vi "project_synthwaveUI.vi"() -> ()   [LabVIEW 2018]
uses:
  <vilib>/sound2/lvsound2.llb/Sampling Mode.ctl
  <vilib>/sound2/lvsound2.llb/Sound Data Format.ctl
  <vilib>/event_ctls.llb/eventvkey.ctl
  <vilib>/sound2/lvsound2.llb/Sound Output Set Volume (Single).vi
  <vilib>/sound2/lvsound2.llb/Sound Output Write (DBL Single).vi
  <vilib>/measure/NI_MABase.lvlib
panel:
  in  "Volume":dbl(knob)=70.40816326530613 scale=0.0..100.0
  in  "Waveform":enum16{"Sine", "Square", "Sawtooth", "Triangle"}(ring)
  out "Generated Sound":waveform(dbl)(graph)
  in  "Keys":T1(radio)=enum."Boolean 1"
  out "Indice":u32
  out "Note Actual":dbl
  in  "?":bool
  in  "Hold Key":bool
  in  "Octave":dbl min=-3.0 max=4.0 step=1.0
  in  "Note Base":dbl=261.626 format="%.2g"
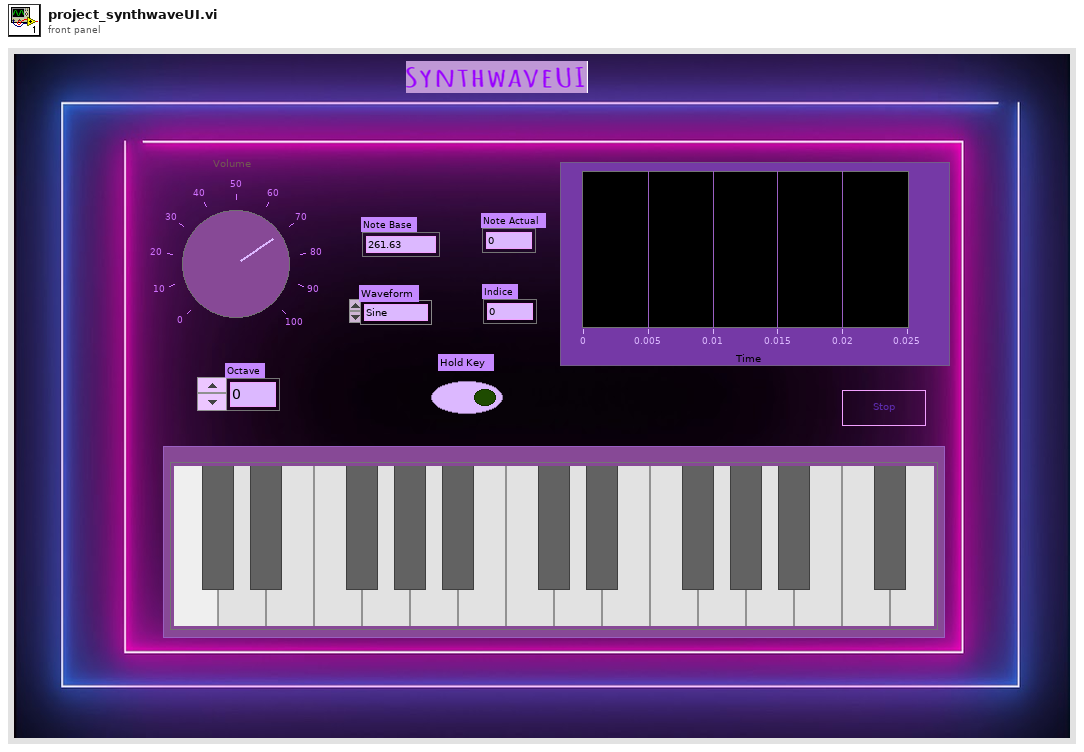
[diagram p1: front panel]
types:
  T1 = enum32{"No Selection", "Boolean 1", "Boolean 2", "Boolean 3", "Boolean 4", "Boolean 5", "Boolean 6", "Boolean 7", "Boolean 8", "Boolean 9", "Boolean 10", "Boolean 11", "Boolean 12", "Boolean 13", "Boolean 14", "Boolean 15", "Boolean 16", "Boolean 17", "Boolean 18", "Boolean 19", "Boolean 20", "Boolean 21", "Boolean 22", "Boolean 23", "Boolean 24", "Boolean 25", "Boolean 26", "Boolean 27"}
  T2 = typedef "eventvkey.ctl" = enum16{"ASCII", "Enter", "Return", "Shift", "Ctrl", "Alt", "Cmd", "Opt", "Caps", "NumLock", "Clear", "Break", "Up", "Down", "Left", "Right", "Insert", "Delete", "Home", "End", "PageUp", "PageDown", "Escape", "Help", "Pause", "ScrollLock", "F1", "F2", "F3", "F4", "F5", "F6", "F7", "F8", "F9", "F10", "F11", "F12", "F13", "F14", "F15", "F16", "F17", "F18", "F19", "F20", "F21", "F22", "F23", "F24", "Play", "VolumeUp", "VolumeDown", "Mute", "Two Byte Char"}
  T3 = typedef "Sound Data Format.ctl" = cluster{"sample rate (S/s)":dbl, "number of channels":i32, "bits per sample":i32}
  T4 = typedef "Sampling Mode.ctl" = i32
  T5 = typedef "Sound Output Task ID.ctl" = u32
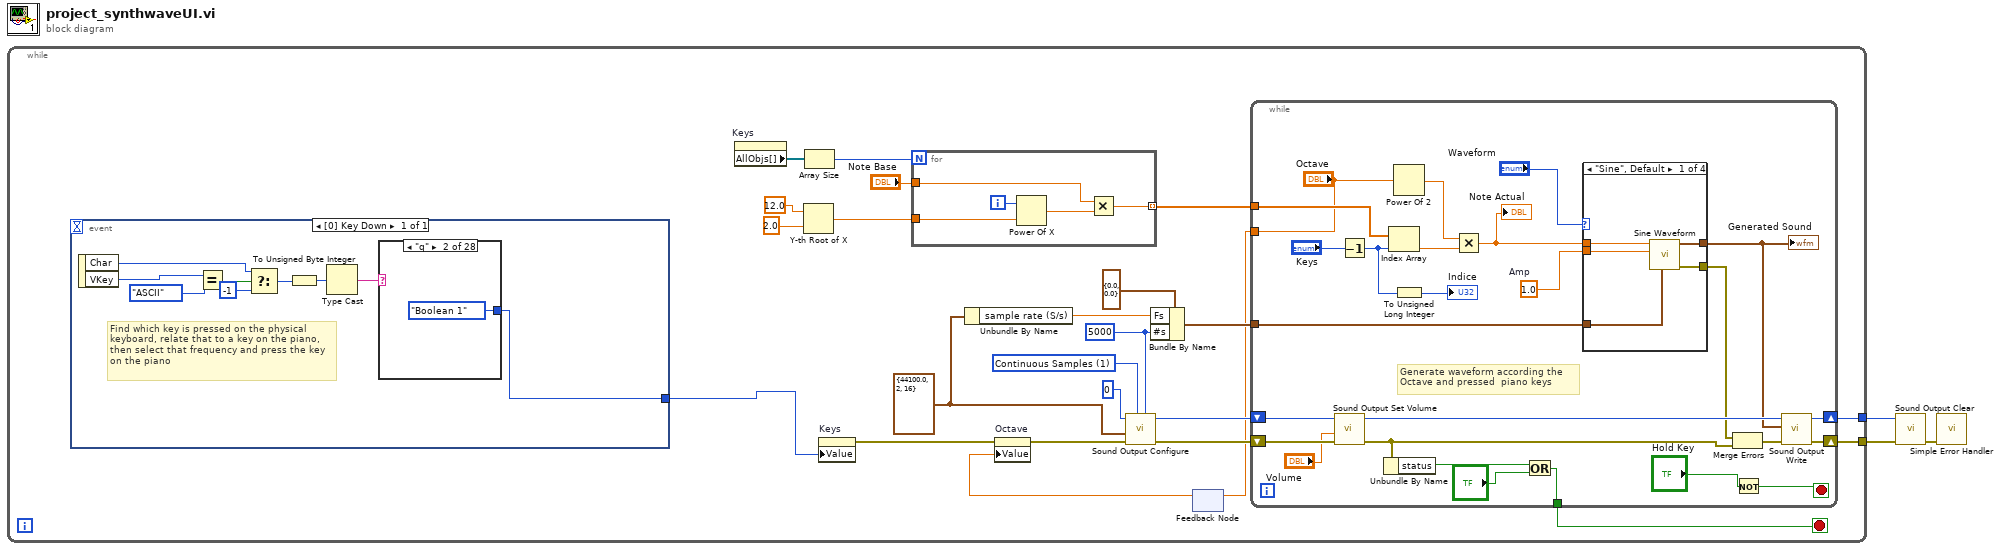
[diagram p0: block diagram]
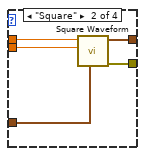
[diagram p2: hidden frame]
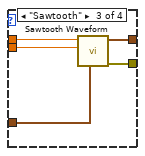
[diagram p3: hidden frame]
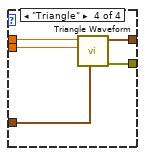
[diagram p4: hidden frame]
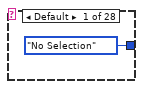
[diagram p5: hidden frame]
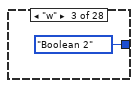
[diagram p6: hidden frame]
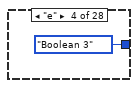
[diagram p7: hidden frame]
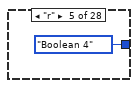
[diagram p8: hidden frame]
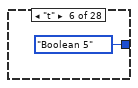
[diagram p9: hidden frame]
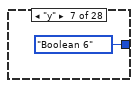
[diagram p10: hidden frame]
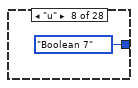
[diagram p11: hidden frame]
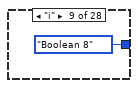
[diagram p12: hidden frame]
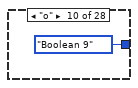
[diagram p13: hidden frame]
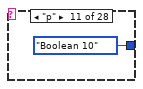
[diagram p14: hidden frame]
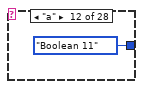
[diagram p15: hidden frame]
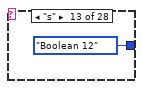
[diagram p16: hidden frame]
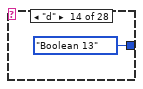
[diagram p17: hidden frame]
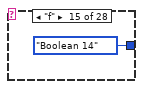
[diagram p18: hidden frame]
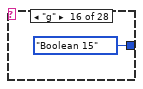
[diagram p19: hidden frame]
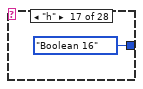
[diagram p20: hidden frame]
diagram:
  n1 = while {
    tunnel: [w27] -> w3
    tunnel: [w26] -> w2
    stop <- w24 stop-if-true
    w12 = 5000 ("Samples/ch")
    w13 = T3 {"sample rate (S/s)"=44100.0, "number of channels"=2, "bits per sample"=16} ("Sound Format")
    w19 = T4 1 items=["Finite Samples", "Continuous Samples"] ("sample mode")
    n2 = event shown="[0] Key Down" {
      selector: _ -> [_]
      dyn-events: _ -> [_]
      timeout: _ -> [_]
      tunnel: [w79] -> w25
      event Key Down {
        # "Find which key is pressed on the physical\nkeyboard, relate that to a key on the piano,\nthen select that frequency and press the key\non the piano"
        n3 = event-data() -> ("Char"=w84:i16, "VKey"=w87:T2)  [unwired: 1 in]
        n4 = Equal?(x=w87, y=eventvkey."ASCII" ("VKey")) -> (x = y?=w85:bool)
        n5 = Select(t=w84, s=w85, f=i16 -1) -> (s? t:f=w81:i16)
        n6 = To Unsigned Byte Integer(number=w81) -> (unsigned 8bit integer=w82:u8)
        n7 = Type Cast(x=w82) -> (*(type *) &x=w80:string)  [unwired: 1 in]
        n8 = case shown="\"q\"" w80 {
          tunnel: [T1."No Selection" ("Keys") T1."Boolean 1" ("Keys") T1."Boolean 2" ("Keys") T1."Boolean 3" ("Keys") T1."Boolean 4" ("Keys") T1."Boolean 5" ("Keys") T1."Boolean 6" ("Keys") T1."Boolean 7" ("Keys") T1."Boolean 8" ("Keys") T1."Boolean 9" ("Keys") T1."Boolean 10" ("Keys") T1."Boolean 11" ("Keys") T1."Boolean 12" ("Keys") T1."Boolean 13" ("Keys") T1."Boolean 14" ("Keys") T1."Boolean 15" ("Keys") T1."Boolean 16" ("Keys") T1."Boolean 17" ("Keys") T1."Boolean 18" ("Keys") T1."Boolean 19" ("Keys") T1."Boolean 20" ("Keys") T1."Boolean 21" ("Keys") T1."Boolean 22" ("Keys") T1."Boolean 23" ("Keys") T1."Boolean 24" ("Keys") T1."Boolean 25" ("Keys") T1."Boolean 26" ("Keys") T1."Boolean 27" ("Keys")] -> w79
          frame Default {
          }
          frame "q" {
          }
          frame "w" {
          }
          frame "e" {
          }
          frame "r" {
          }
          frame "t" {
          }
          frame "y" {
          }
          frame "u" {
          }
          frame "i" {
          }
          frame "o" {
          }
          frame "p" {
          }
          frame "a" {
          }
          frame "s" {
          }
          frame "d" {
          }
          frame "f" {
          }
          frame "g" {
          }
          frame "h" {
          }
          frame "j" {
          }
          frame "k" {
          }
          frame "l" {
          }
          frame ";" {
          }
          frame "z" {
          }
          frame "x" {
          }
          frame "c" {
          }
          frame "v" {
          }
          frame "b" {
          }
          frame "n" {
          }
          frame "m" {
          }
        }
      }
    }
    n9 = property on="Keys" class="RadioBtnsControl (strict)"() -> ("AllObjs[]"=w15:refnum<vi>[])  [unwired: 2 in, 2 out]
    n10 = Y-th Root of X(1:2.0 ("x"), 2:12.0 ("y")) -> (0:w8:dbl)
    n11 = Array Size(array=w15) -> (size(s)=w14:i32)
    n12 = property on="Keys" class="RadioBtnsControl (strict)"("Value"=w25) -> (error out=w7:errorcluster)  [unwired: 2 in, 1 out]
    n13 = for {
      N: w14 -> [_]
      tunnel: [w32] -> w20 mode=indexing
      tunnel: "Note Base" -> [w31]
      tunnel: w8 -> [w28]
      i -> [w30]
      n14 = Power Of X(1:w28, 2:w30) -> (0:w29:dbl)
      n15 = Multiply(x=w31, y=w29) -> (x*y=w32:dbl)
    }
    n16 = Unbundle By Name(w13) -> ("sample rate (S/s)"=w17:dbl)
    n17 = Bundle By Name(cluster=cluster{"Fs":dbl, "#s":dbl} {"Fs"=0.0, "#s"=0.0} ("sampling info"), "Fs"=w17, "#s"=w12) -> (w21:cluster{"Fs":dbl, "#s":dbl})
    n18 = feedback #1() -> (w4:dbl)  [unwired: 1 in]
    n19 = property on="Octave" class="DigNum (strict)"(error in=w7, "Value"=w4) -> (error out=w6:errorcluster)  [unwired: 1 in, 1 out]
    n20 = call <vilib>:"Sound Output Configure.vi"("number of samples/ch"=w12, "sample mode"=w19, "error in (no error)"=w6, "sound format"=w13, "device ID"=u32 0 ("Device ID")) -> ("error out"=w23:errorcluster, "task ID"=w22:T5)  [unwired: 5 in]
    n21 = while {
      tunnel: [w56] -> w24
      tunnel: w21 -> [w53]
      tunnel: w20 -> [w52]
      shift-right: [w58] -> w27
      shift-left: w23 -> [w55]
      shift-right: [w57] -> w26
      shift-left: w22 -> [w54]
      tunnel: ["Octave"] -> w5
      stop <- w33 stop-if-true
      w46 = 1.0  # Amp
      # "Generate waveform according the \nOctave and pressed  piano keys"
      n22 = call-poly <vilib>:"Sound Output Set Volume.vi"("error in (no error)"=w55, "volume"="Volume", "task ID"=w54) -> ("error out"=w49:errorcluster, "task ID out"=w51:T5)  [unwired: 7 in]
      n23 = Decrement(x="Keys") -> (x-1=w43:T1)
      n24 = Unbundle By Name(w49) -> ("status"=w48:bool)
      n25 = Index Array(array=w52, index=w43) -> (element=w41:dbl)
      n26 = Power Of 2(x="Octave") -> (2^x=w39:dbl)
      n27 = To Unsigned Long Integer(number=w43) -> (unsigned 32bit integer=→"Indice":u32)
      n28 = Multiply(x=w39, y=w41) -> (x*y=w40:dbl)
      "Note Actual" <- w40
      n29 = Or(x=w48, y="?") -> (x .or. y?=w56:bool)
      n30 = case shown="\"Sine\", Default" "Waveform" {
        tunnel: [w63 w67 w72 w78] -> w42
        tunnel: w53 -> [w62 w68 w73 w77]
        tunnel: w46 -> [w61 w66 w71 w76]
        tunnel: w40 -> [w60 w65 w70 w75]
        tunnel: [w59 w64 w69 w74] -> w38
        frame "Sine", Default {
          n31 = call <vilib>:"Sine Waveform.vi"("sampling info"=w62, "amplitude"=w61, "frequency"=w60) -> ("error out"=w59:errorcluster, "signal out"=w63:waveform(dbl))  [unwired: 7 in]
        }
        frame "Square" {
          n32 = call <vilib>:"Square Waveform.vi"("sampling info"=w68, "amplitude"=w66, "frequency"=w65) -> ("error out"=w64:errorcluster, "signal out"=w67:waveform(dbl))  [unwired: 7 in]
        }
        frame "Sawtooth" {
          n33 = call <vilib>:"Sawtooth Waveform.vi"("sampling info"=w73, "amplitude"=w71, "frequency"=w70) -> ("error out"=w69:errorcluster, "signal out"=w72:waveform(dbl))  [unwired: 7 in]
        }
        frame "Triangle" {
          n34 = call <vilib>:"Triangle Waveform.vi"("sampling info"=w77, "amplitude"=w76, "frequency"=w75) -> ("error out"=w74:errorcluster, "signal out"=w78:waveform(dbl))  [unwired: 7 in]
        }
      }
      "Generated Sound" <- w42
      n35 = Merge Errors(w38, w49) -> (w37:errorcluster)
      n36 = Not(x="Hold Key") -> (.not. x?=w33:bool)
      n37 = call-poly <vilib>:"Sound Output Write.vi"("error in (no error)"=w37, "data"=w42, "task ID"=w51) -> ("error out"=w58:errorcluster, "task ID out"=w57:T5)  [unwired: 7 in]
    }
    n38 = feedback-in #1(w5) -> ()
  }
  n39 = call <vilib>:"Sound Output Clear.vi"("error in (no error)"=w3, "task ID"=w2) -> ("error out"=w1:errorcluster)  [unwired: 9 in]
  n40 = call <vilib>:"Simple Error Handler.vi"("error in (no error)"=w1) -> ()  [unwired: 4 in, 5 out]
